vi "Page - Line.vi"(8 "error in (no error)":errorcluster, 11 "Node Ptr":T2 format="%.0x") -> (0 "error out":errorcluster)   [LabVIEW 2015, in "SLSC-12201 DIO System Explorer.lvlib"]
uses:
  SLSC-12201 DIO System Explorer.lvlib
  <vilib>/NI Veristand/Custom Device API/Custom Device Item Ref.ctl
  Direction Control.ctl
  Shared/Constants.vi
  <vilib>/NI Veristand/Custom Device API/Custom Device API.lvlib
  Shared/SLSC-12201 DIO Shared.lvlib
panel:
  out "Index":i32
  in  "*Enable":bool
  in  "*Direction":T1 caption="Type" items=["Input", "Output Source", "Output Sink", "Output Push-Pull"]
  in  "SHDocVw.IWebBrowser2":refnum<k7>(container)
  in  "Header":cluster{"Section Name":string}={"Section Name"="Custom Device Item Settings"}
  in  "Description":string
  out "Name":string
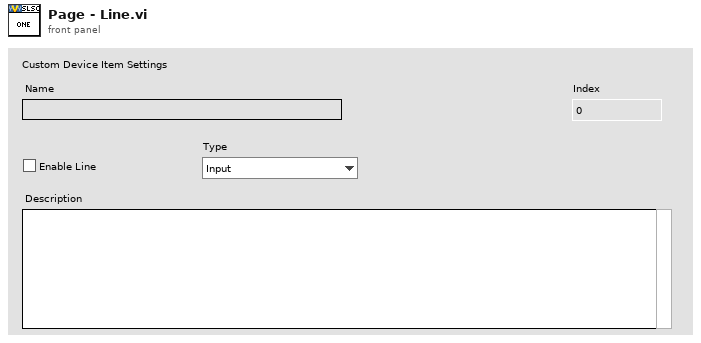
[diagram p1: front panel]
types:
  T1 = typedef "SLSC-12201 DIO System Explorer.lvlib/Direction Control.ctl" = u16
  T2 = typedef "Custom Device API.lvlib/Custom Device Item Ref.ctl" = u64
  T3 = typedef "Custom Device API.lvlib/Custom Device Channel.ctl" = cluster{"Type":T4, "Units":string, "Default Value":dbl, "Faultable":bool, "Scalable":bool}
  T4 = typedef "Custom Device API.lvlib/Custom Device Channel Type.ctl" = enum16{"Input", "Output"}
  T5 = cluster{"Channel Name":string, "SLSC Name":string, "Channel":T3}[]
  T6 = typedef "Custom Device API.lvlib/Custom Device Item Info.ctl" = cluster{"Name":string, "Is Channel":bool, "GUID":string, "Is Waveform":bool}
  T7 = typedef "Custom Device API.lvlib/Custom Device Commands.ctl" = enum16{"Default", "Item renamed", "Shutdown", "Dynamic button pressed"}
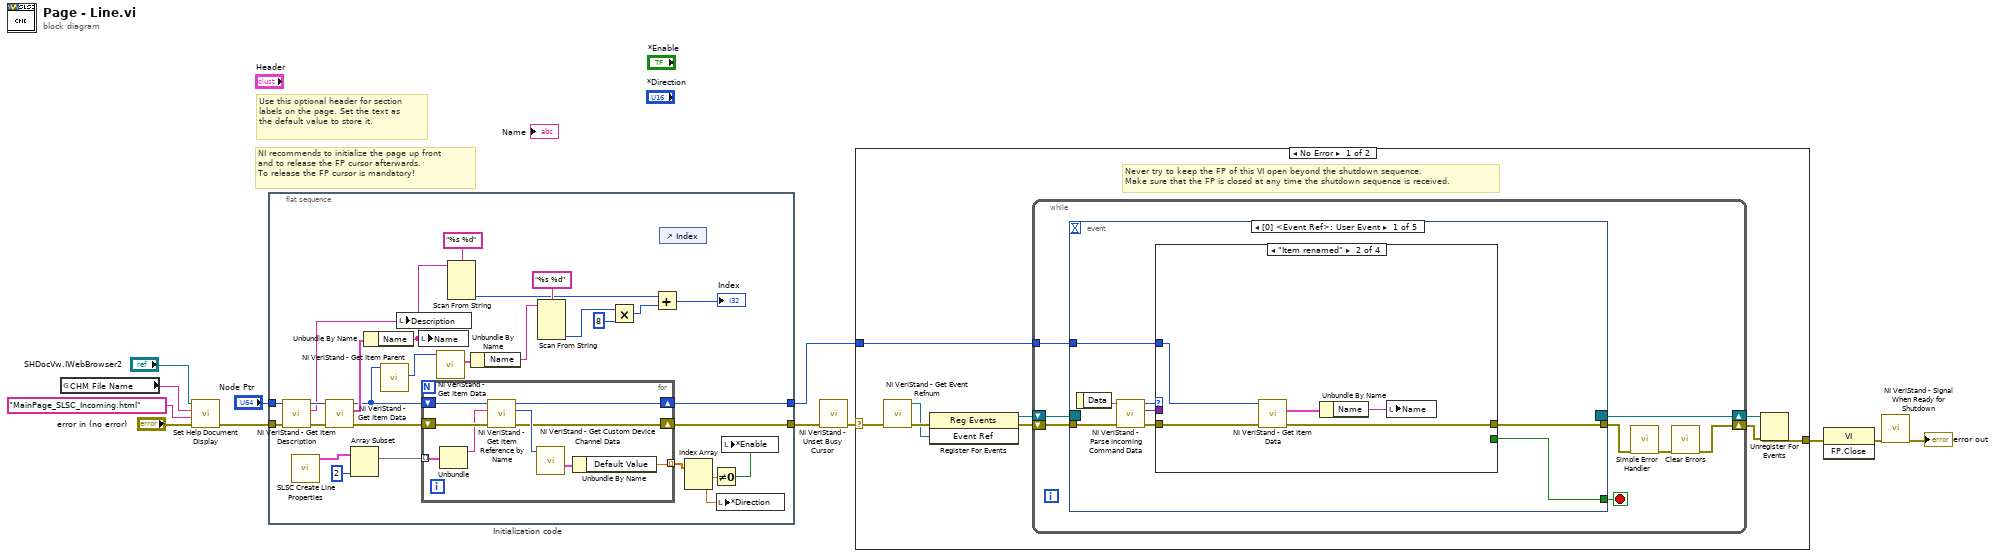
[diagram p0: block diagram]
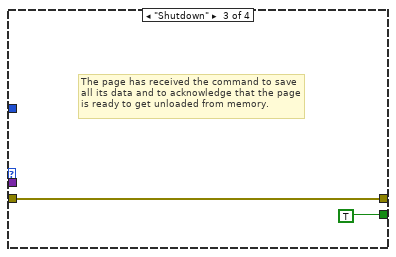
[diagram p3: hidden frame]
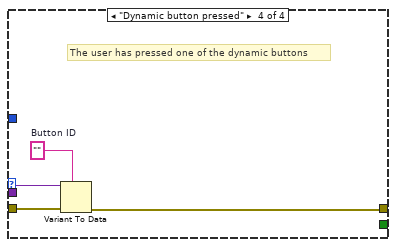
[diagram p4: hidden frame]
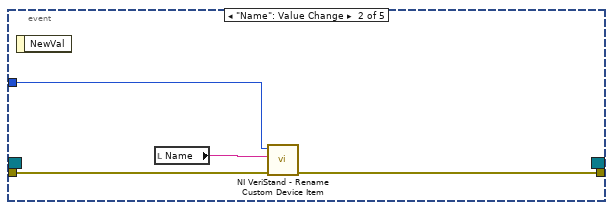
[diagram p5: hidden frame]
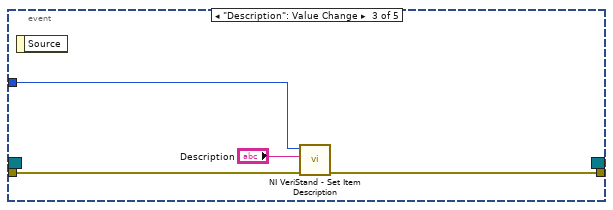
[diagram p6: hidden frame]
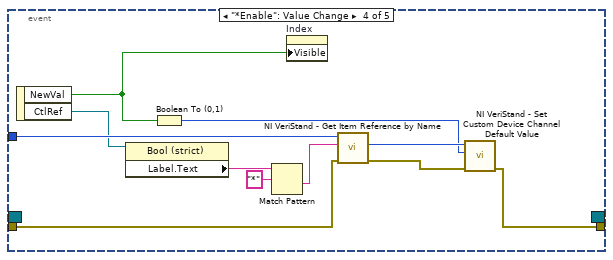
[diagram p7: hidden frame]
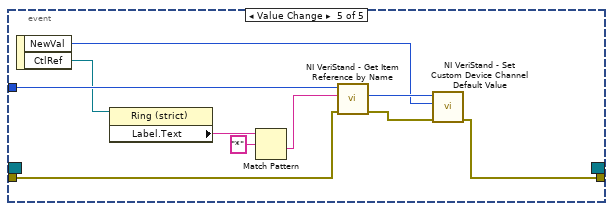
[diagram p8: hidden frame]
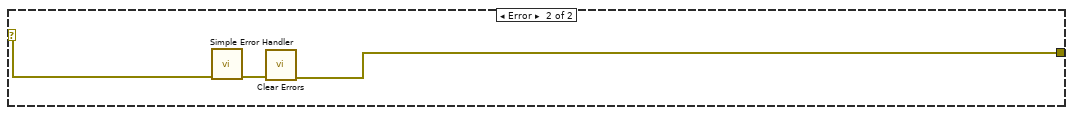
[diagram p9: hidden frame]
diagram:
  # "Use this optional header for section labels on the page. Set the text as the default value to store it."
  # "NI recommends to initialize the page up front\nand to release the FP cursor afterwards.\nTo release the FP cursor is mandatory!"
  n1 = global read "Constants.vi" "CHM File Name"() -> (w1:string)
  n2 = call "Set Help Document Display.vi"("error in (no error)"="error in (no error)", "HTML File"="MainPage_SLSC_Incoming.html", "Main CHM File"=w1, "SHDocVw.IWebBrowser2"="SHDocVw.IWebBrowser2") -> ("error out"=w2:errorcluster)  [unwired: 7 in]
  n3 = flat-sequence "Initialization code" {
    tunnel: w2 -> [w39]
    tunnel: "Node Ptr" -> [w38]
    tunnel: [w33] -> w8
    tunnel: [w32] -> w6
    frame #0 {
      n4 = call <vilib>:"NI VeriStand - Get Item Description.vi"("error in (no error)"=w39, "Item Ref in"=w38) -> ("error out"=w36:errorcluster, "Description"=w37:string, "Item Ref out"=w40:T2)  [unwired: 7 out]
      n5 = call "SLSC Create Line Properties.vi"() -> ("Outgoing configuration"=w31:T5)  [unwired: 11 in]
      n6 = call <vilib>:"NI VeriStand - Get Item Data.vi"("error in (no error)"=w36, "Item Ref in"=w40) -> ("error out"=w34:errorcluster, "Item Info"=w35:T6, "Item Ref out"=w26:T2)  [unwired: 7 out]
      n7 = Array Subset(array=w31, length=2) -> (w30:T5)  [unwired: 1 in]
      n8 = Unbundle By Name(w35) -> ("Name"=w27:string)
      n9 = call <vilib>:"NI VeriStand - Get Item Parent.vi"("Item Ref in"=w26) -> ("Parent Ref"=w25:T2)  [unwired: 7 in, 3 out]
      n10 = local write "Description"(w37) -> ()
      n11 = local write "Name"(w27) -> ()
      n12 = for {
        shift-right: [w46] -> w33
        shift-left: w34 -> [w47]
        shift-right: [w44] -> w32
        shift-left: w26 -> [w45]
        tunnel: w30 -> [w43] mode=indexing
        tunnel: [w41] -> w16 mode=indexing
        n13 = Unbundle(w43) -> ("Channel Name"=w42:string)  [unwired: 2 out]
        n14 = call <vilib>:"NI VeriStand - Get Item Reference by Name.vi"("error in (no error)"=w47, "Item Name"=w42, "Parent Ref in"=w45) -> ("error out"=w46:errorcluster, "Item Ref"=w49:T2, "Parent Ref out"=w44:T2)  [unwired: 5 in, 1 out]
        n15 = call <vilib>:"NI VeriStand - Get Custom Device Channel Data.vi"("Channel Ref in"=w49) -> ("Channel"=w48:T3)  [unwired: 5 in, 5 out]
        n16 = Unbundle By Name(w48) -> ("Default Value"=w41:dbl)
      }
      n17 = call <vilib>:"NI VeriStand - Get Item Data.vi"("Item Ref in"=w25) -> ("Item Info"=w24:T6)  [unwired: 1 in, 9 out]
      n18 = Scan From String(format string="%s %d", input string=w27) -> (output 2=w18:i32)  [unwired: 5 in, 3 out]
      n19 = Unbundle By Name(w24) -> ("Name"=w22:string)
      n20 = Scan From String(format string="%s %d", input string=w22) -> (output 2=w21:i32)  [unwired: 5 in, 3 out]
      n21 = Multiply(x=w21, y=8) -> (x*y=w19:i32)
      n22 = Add(x=w18, y=w19) -> (x+y=→"Index":i32)
      n23 = control-ref of="Index"() -> ()  [unwired: 1 out]
      n24 = Index Array(array=w16) -> (element #1=w15:dbl, element #2=w13:dbl)  [unwired: 2 in]
      n25 = Not Equal To 0?(x=w15) -> (x != 0?=w14:bool)
      n26 = local write "*Direction"(w13) -> ()
      n27 = local write "*Enable"(w14) -> ()
    }
  }
  n28 = call <vilib>:"NI VeriStand - Unset Busy Cursor.vi"("error in (no error)"=w8) -> ("error out"=w7:errorcluster)  [unwired: 10 out]
  n29 = case shown="No Error" w7 {
    selector: w7 -> [w50 w118]
    tunnel: [w55 w116] -> w12
    tunnel: w6 -> [w51 _]
    frame No Error {
      # "Never try to keep the FP of this VI open beyond the shutdown sequence.\nMake sure that the FP is closed at any time the shutdown sequence is received."
      n30 = call <vilib>:"NI VeriStand - Get Event Refnum.vi"("error in (no error)"=w50) -> ("error out"=w58:errorcluster, "Event Ref"=w54:refnum<user-event>)  [unwired: 9 out]
      n31 = register-events(error in=w58, w54) -> (reference out=w52:refnum<event-registration>, error out=w53:errorcluster)  [unwired: 1 in]
      n32 = while {
        tunnel: w51 -> [w62]
        shift-right: [w59] -> w56
        shift-left: w53 -> [w65]
        shift-right: [w66] -> w57
        shift-left: w52 -> [w64]
        stop <- w63 stop-if-true
        n33 = event shown="[0] <Event Ref>: User Event" {
          selector: w64 -> [_ _ _ _ _]
          dyn-events: [_ _ _ _ _] -> w66
          timeout: _ -> [_ _ _ _ _]
          tunnel: w65 -> [w74 w90 w93 w102 w113]
          tunnel: [w70 _ _ _ _] -> w63
          tunnel: [w69 w89 w92 w100 w111] -> w61
          tunnel: w62 -> [w68 w88 w94 w105 w115]
          event User Event {
            n34 = event-data() -> ("Data"=w73:string)  [unwired: 1 out]
            n35 = call <vilib>:"NI VeriStand - Parse Incoming Command Data.vi"("error in (no error)"=w74, "Incoming data"=w73) -> ("error out"=w72:errorcluster, "Outgoing data"=w67:variant, "Action"=w71:T7)  [unwired: 7 out]
            n36 = case shown="\"Item renamed\"" w71 {
              tunnel: w72 -> [w75 w80 w81 w86]
              tunnel: [_ _ TRUE _] -> w70
              tunnel: [w75 w77 w81 w83] -> w69
              tunnel: w68 -> [_ w79 _ _]
              tunnel: w67 -> [_ _ _ w85]
              frame "Default", Default {
              }
              frame "Item renamed" {
                n37 = call <vilib>:"NI VeriStand - Get Item Data.vi"("error in (no error)"=w80, "Item Ref in"=w79) -> ("error out"=w77:errorcluster, "Item Info"=w78:T6)  [unwired: 8 out]
                n38 = Unbundle By Name(w78) -> ("Name"=w76:string)
                n39 = local write "Name"(w76) -> ()
              }
              frame "Shutdown" {
                # "The page has received the command to save all its data and to acknowledge that the page is ready to get unloaded from memory."
              }
              frame "Dynamic button pressed" {
                w84 = ""  # Button ID
                # "The user has pressed one of the dynamic buttons"
                n40 = Variant To Data(error in=w86, type=w84, Variant=w85) -> (error out=w83:errorcluster)  [unwired: 1 out]
              }
            }
          }
          event "Name": Value Change {
            n41 = event-data() -> ()  [unwired: 2 out]
            n42 = local read "Name"() -> (w87:string)
            n43 = call <vilib>:"NI VeriStand - Rename Custom Device Item.vi"("error in (no error)"=w90, "New Name"=w87, "Item Ref in"=w88) -> ("error out"=w89:errorcluster)  [unwired: 1 in, 7 out]
          }
          event "Description": Value Change {
            n44 = event-data() -> ()  [unwired: 2 out]
            n45 = call <vilib>:"NI VeriStand - Set Item Description.vi"("error in (no error)"=w93, "Description"="Description", "Item Ref in"=w94) -> ("error out"=w92:errorcluster)  [unwired: 8 out]
          }
          event "*Enable": Value Change {
            n46 = event-data() -> ("NewVal"=w95:bool, "CtlRef"=w97:refnum<vi>)  [unwired: 1 out]
            n47 = property class="Bool (strict)"(reference=w97) -> ("Label.Text"=w99:string)  [unwired: 1 in, 2 out]
            n48 = Boolean To (0,1)(Boolean=w95) -> (0, 1=w103:i16)
            n49 = Match Pattern(string=w99, regular expression="*") -> (after substring=w96:string)  [unwired: 1 in, 3 out]
            n50 = property on="Index" class="DigNum (strict)"("Visible"=w95) -> ()  [unwired: 2 in, 2 out]
            n51 = call <vilib>:"NI VeriStand - Get Item Reference by Name.vi"("error in (no error)"=w102, "Item Name"=w96, "Parent Ref in"=w105) -> ("error out"=w101:errorcluster, "Item Ref"=w104:T2)  [unwired: 5 in, 2 out]
            n52 = call <vilib>:"NI VeriStand - Set Custom Device Channel Default Value.vi"("error in (no error)"=w101, "Default Value"=w103, "Channel Ref in"=w104) -> ("error out"=w100:errorcluster)  [unwired: 7 in, 1 out]
          }
          event Value Change {
            n53 = event-data() -> ("NewVal"=w106:T1, "CtlRef"=w110:refnum<vi>)  [unwired: 1 out]
            n54 = property class="Ring (strict)"(reference=w110) -> ("Label.Text"=w109:string)  [unwired: 1 in, 2 out]
            n55 = Match Pattern(string=w109, regular expression="*") -> (after substring=w107:string)  [unwired: 1 in, 3 out]
            n56 = call <vilib>:"NI VeriStand - Get Item Reference by Name.vi"("error in (no error)"=w113, "Item Name"=w107, "Parent Ref in"=w115) -> ("error out"=w112:errorcluster, "Item Ref"=w114:T2)  [unwired: 5 in, 2 out]
            n57 = call <vilib>:"NI VeriStand - Set Custom Device Channel Default Value.vi"("error in (no error)"=w112, "Default Value"=w106, "Channel Ref in"=w114) -> ("error out"=w111:errorcluster)  [unwired: 7 in, 1 out]
          }
        }
        n58 = call <vilib>:"Simple Error Handler.vi"("error in (no error)"=w61) -> ("error out"=w60:errorcluster)  [unwired: 1 in, 7 out]
        n59 = call <vilib>:"Clear Errors.vi"("error in (no error)"=w60) -> ("error out"=w59:errorcluster)  [unwired: 1 in, 5 out]
      }
      n60 = Unregister For Events(event registration refnum=w57, error in=w56) -> (error out=w55:errorcluster)
    }
    frame Error {
      n61 = call <vilib>:"Simple Error Handler.vi"("error in (no error)"=w118) -> ("error out"=w117:errorcluster)  [unwired: 1 in, 7 out]
      n62 = call <vilib>:"Clear Errors.vi"("error in (no error)"=w117) -> ("error out"=w116:errorcluster)  [unwired: 1 in, 5 out]
    }
  }
  n63 = invoke class="VI" method="FP.Close"(error in=w12) -> (error out=w11:errorcluster)  [unwired: 2 in, 2 out]
  n64 = call <vilib>:"NI VeriStand - Signal When Ready for Shutdown.vi"("error in (no error)"=w11) -> ("error out"=→"error out":errorcluster)  [unwired: 10 out]
